vi "TestStaleInsertIntoPanel_Reject.vi"(8 "error in (no error)":errorcluster, 11 "TestCase in":refnum<class "TestProtectedSubpanel.lvclass">) -> (0 "error out":errorcluster, 3 "TestCase out":refnum<class "TestProtectedSubpanel.lvclass">)   [LabVIEW 2017, in "TestProtectedSubpanel.lvclass"]
uses:
  TestProtectedSubpanel.lvclass
  TestProtectedSubpanel.lvclass/TestProtectedSubpanel.ctl
  IViewable/IViewable.lvclass/IViewable.ctl
  ProtectedSubpanel/ProtectedSubpanel.lvclass/ProtectedSubpanel.ctl
  ProtectedSubpanel/Evaluate Insertion Request.vi
  IViewable/Evaluate Destination Subpanel.vi
  ProtectedSubpanel/Do Insertion.vi
  IViewable/IViewable.lvclass
  ProtectedSubpanel/ProtectedSubpanel.lvclass
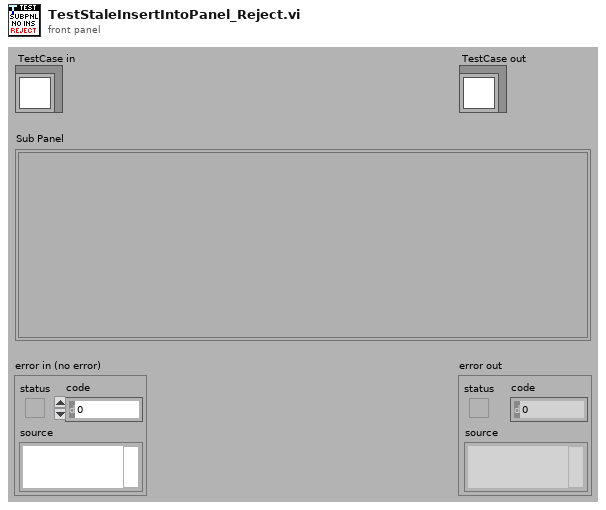
[diagram p1: front panel]
types:
  T1 = typedef "IViewable.lvlib/ProtectedSubpanel.lvclass/Protected Subpanel Reference.ctl" = refnum<data-value>
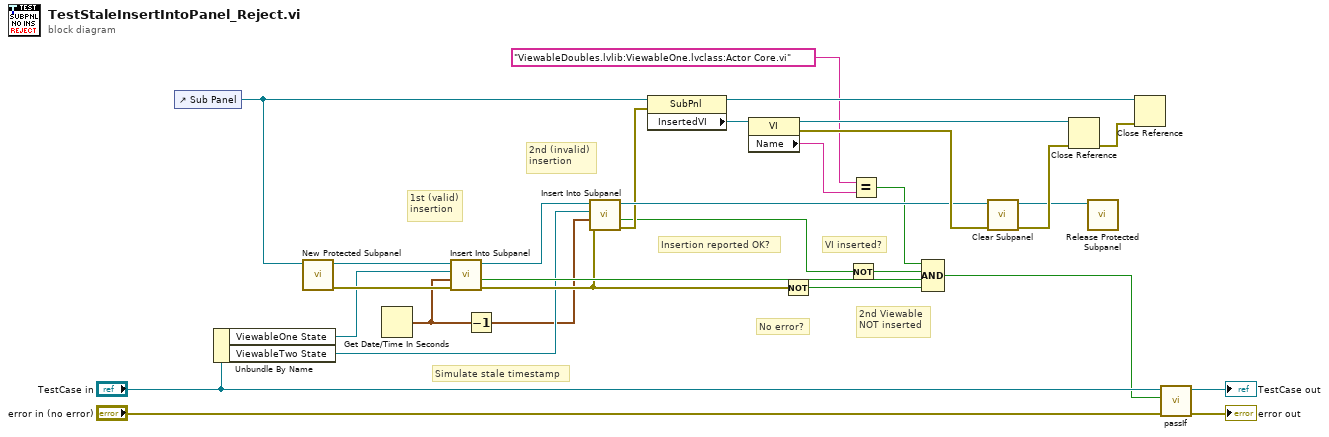
[diagram p0: block diagram]
diagram:
  # "2nd Viewable\nNOT inserted"
  # "Simulate stale timestamp"
  # "2nd (invalid)\ninsertion"
  # "1st (valid)\ninsertion"
  # "Insertion reported OK?"
  # "No error?"
  # "VI inserted?"
  n1 = control-ref of="Sub Panel"() -> (w1:refnum<vi>)
  n2 = Unbundle By Name("TestCase in") -> ("ViewableOne State"=w19:refnum<class "IViewable.lvclass">, "ViewableTwo State"=w9:refnum<class "IViewable.lvclass">)
  n3 = call "New Protected Subpanel.vi"("SubPnl Refnum"=w1) -> ("error out"=w23:errorcluster, "Protected Subpanel"=w30:T1)  [unwired: 9 in]
  n4 = Get Date/Time In Seconds() -> (seconds since 1Jan1904=w8:timestamp)
  n5 = call "Insert Into Subpanel.vi"("error in (no error)"=w23, "Insertion Request Time"=w8, "Viewable"=w19, "Protected Subpanel"=w30) -> ("error out"=w10:errorcluster, "Inserted?"=w22:bool, "Protected Subpanel"=w24:T1)  [unwired: 4 in, 1 out]
  n6 = Decrement(x=w8) -> (x-1=w7:timestamp)
  n7 = call "Insert Into Subpanel.vi"("error in (no error)"=w10, "Insertion Request Time"=w7, "Viewable"=w9, "Protected Subpanel"=w24) -> ("error out"=w6:errorcluster, "Inserted?"=w3:bool, "Protected Subpanel"=w11:T1)  [unwired: 4 in, 1 out]
  n8 = property class="SubPnl"(reference=w1, error in=w6) -> (reference out=w26:refnum<vi>, "InsertedVI"=w28:refnum<vi>)  [unwired: 1 out]
  n9 = property class="VI"(reference=w28) -> (reference out=w21:refnum<vi>, error out=w18:errorcluster, "Name"=w27:string)  [unwired: 1 in]
  n10 = Not(x=w10) -> (.not. x?=w29:bool)
  n11 = Not(x=w3) -> (.not. x?=w4:bool)
  n12 = Equal?(x="ViewableDoubles.lvlib:ViewableOne.lvclass:Actor Core.vi" ("y"), y=w27) -> (x = y?=w5:bool)
  n13 = Compound Arithmetic op=AND(w5, w4, w22, w29) -> (w12:bool)
  n14 = call "Clear Subpanel.vi"("error in (no error)"=w18, "Protected Subpanel"=w11) -> ("error out"=w20:errorcluster, "Protected Subpanel Out"=w2:T1)  [unwired: 8 in]
  n15 = Close Reference(reference=w21, error in (no error)=w20) -> (error out=w25:errorcluster)
  n16 = call "Release Protected Subpanel.vi"("Protected Subpanel"=w2) -> ()  [unwired: 10 in, 1 out]
  n17 = Close Reference(reference=w26, error in (no error)=w25) -> ()  [unwired: 1 out]
  n18 = call-dynamic "passIf.vi"("error in (no error)"="error in (no error)", "pass"=w12, "TestCase in"="TestCase in") -> ("error out"=→"error out":errorcluster, "TestCase out"=→"TestCase out":refnum<class "TestProtectedSubpanel.lvclass">)  [unwired: 7 in]
